vi "Load Config.vi"(6 "Constants":refnum<class "Sequence Constants.lvclass">, 8 "error in (no error)":refnum<class "MultiErrors.lvclass">, 10 "Config Element":refnum<class "Config Element.lvclass">, 11 "Error Command Config in":refnum<class "Error Command Config.lvclass">) -> (0 "error out":refnum<class "MultiErrors.lvclass">, 3 "Error Command Config out":refnum<class "Error Command Config.lvclass">)   [LabVIEW 2020, in "VolatusSeqConfig.lvlib" / "Error Command Config.lvclass"]
uses:
  Error Command Config.lvclass
  VolatusErrorUtilities/MultiErrors/MultiErrors.lvclass
  lv-cdm/CDM-Config/Config Element/Config Element.lvclass
  Error Command Config.lvclass/Error Command Config.ctl
  Sequence Constants/Sequence Constants.lvclass
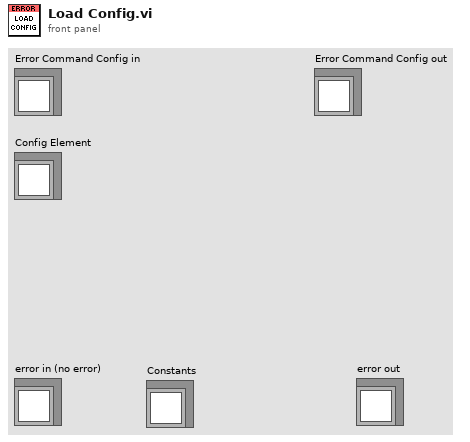
[diagram p1: front panel]
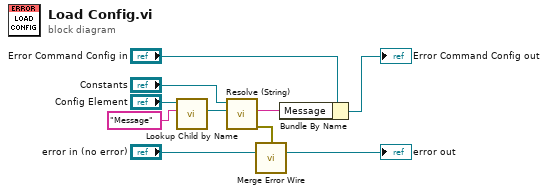
[diagram p0: block diagram]
diagram:
  n1 = call "Lookup Child by Name.vi"("Name"="Message", "Config Element in"="Config Element") -> ("Child"=w4:refnum<class "Config Element.lvclass">)  [unwired: 6 in, 3 out]
  n2 = call "Resolve (String).vi"("Element"=w4, "Sequence Constants in"="Constants") -> ("error out"=w1:errorcluster, "String Value"=w2:string)  [unwired: 7 in, 1 out]
  n3 = call "Merge Error Wire.vi"("error in (no error)"=w1, "MultiErrors in"="error in (no error)") -> ("MultiErrors out"=→"error out":refnum<class "MultiErrors.lvclass">)  [unwired: 13 in]
  n4 = Bundle By Name(cluster="Error Command Config in", "Message"=w2) -> (→"Error Command Config out":refnum<class "Error Command Config.lvclass">)
